vi "Motion_subsystem.vi"(10 "Parameters":dbl[](array[numeric]), 11 "ControlWord":u16 format="%.0b") -> (2 "Results":dbl[](array[numeric]), 3 "StatusWord":u16, 4 "Enum":T1)   [LabVIEW 2017]
uses:
  Utilities/StateMachine.ctl
  SoftmotionAxis/SoftmotionAxis.lvclass
  Utilities/Controlword_Commands.ctl
  Utilities/Mode.ctl
  Utilities/WordManipulationLibrary.lvlib
  Utilities/Bit Manipulation.lvlib
panel:
  out "error out":errorcluster
  in  "error in":errorcluster
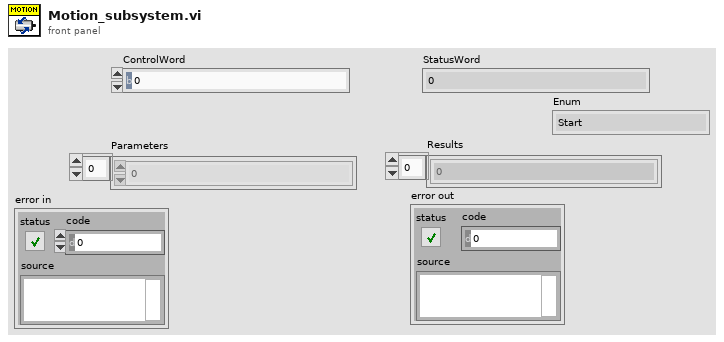
[diagram p1: front panel]
types:
  T1 = typedef "WordManipulationLibrary.lvlib/StateMachine.ctl" = enum16{"Start", "Not Ready to Switch On", "Switch On Disabled", "Ready to Switch On", "Switched On", "Operation enable", "Quick Stop Active", "Fault Reaction Active", "Fault"}
  T2 = typedef "WordManipulationLibrary.lvlib/Controlword_Commands.ctl" = enum16{"Shutdown", "Switch On", "Disable Voltage", "Quick Stop", "Disable Op", "Enable Op", "Fault Reset", "Error"}
  T3 = typedef "WordManipulationLibrary.lvlib/Mode.ctl" = enum16{"Reserved", "Profile Position Mode", "Velocity Mode", "Profile Velocity Mode", "Profile Torque Mode", "Reserved 2", "Reference Mode", "Interpolated Position Mode", "Skip"}
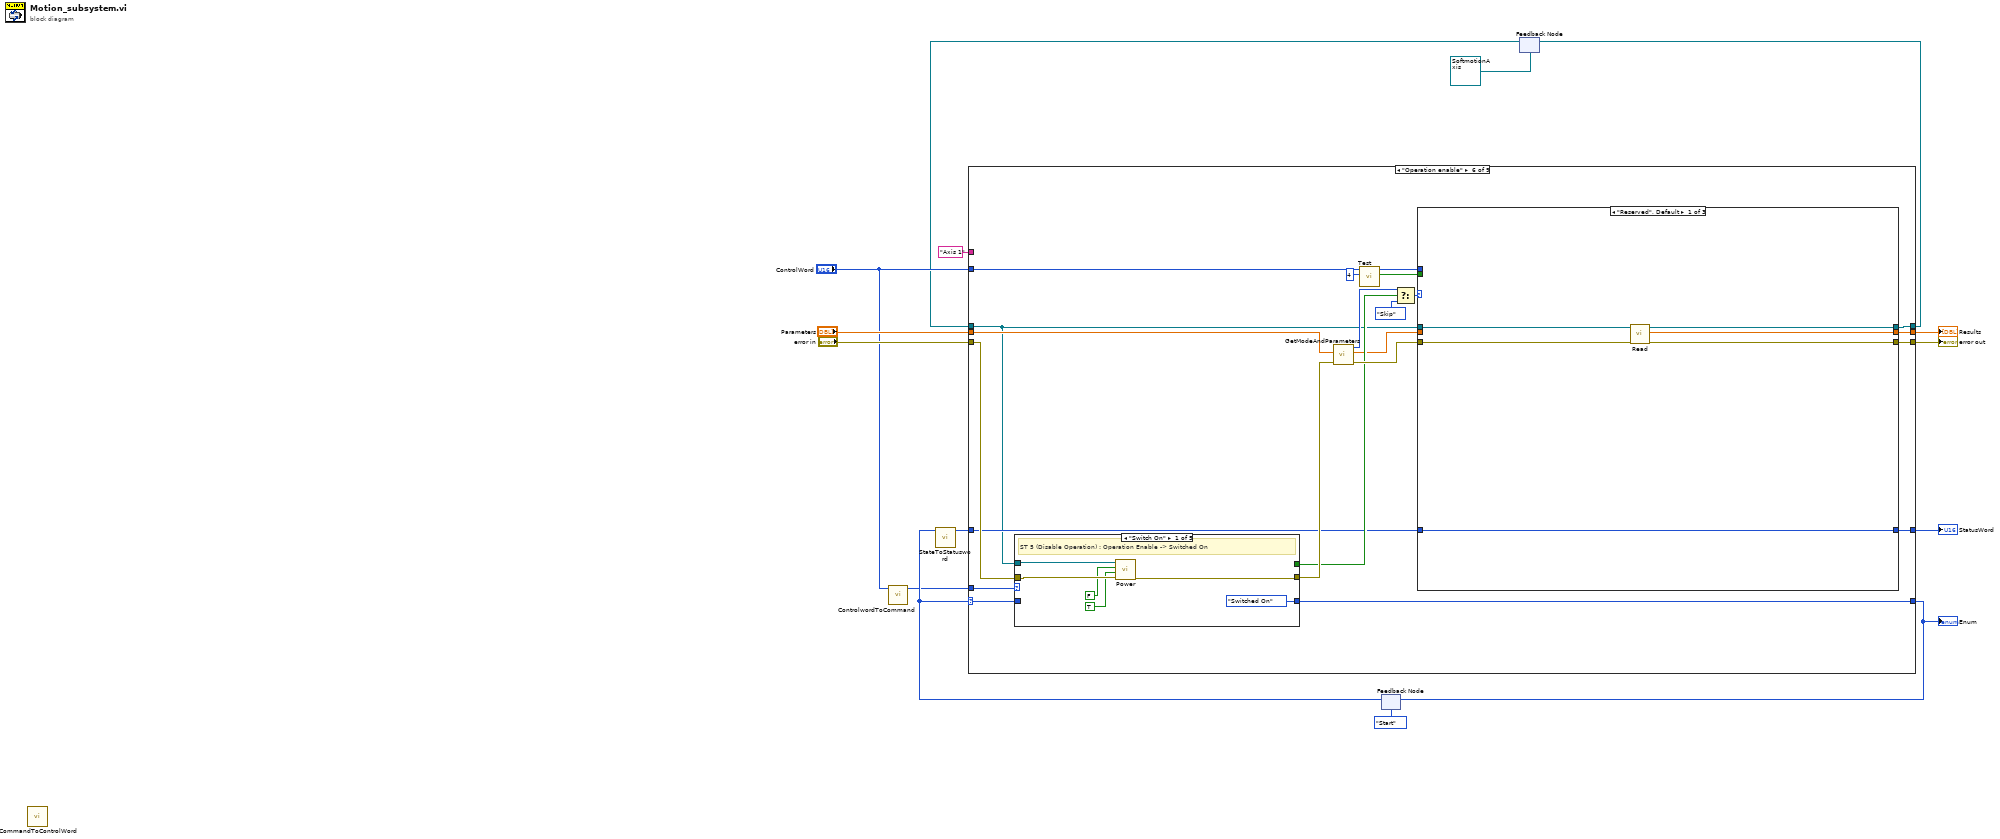
[diagram p0: block diagram]
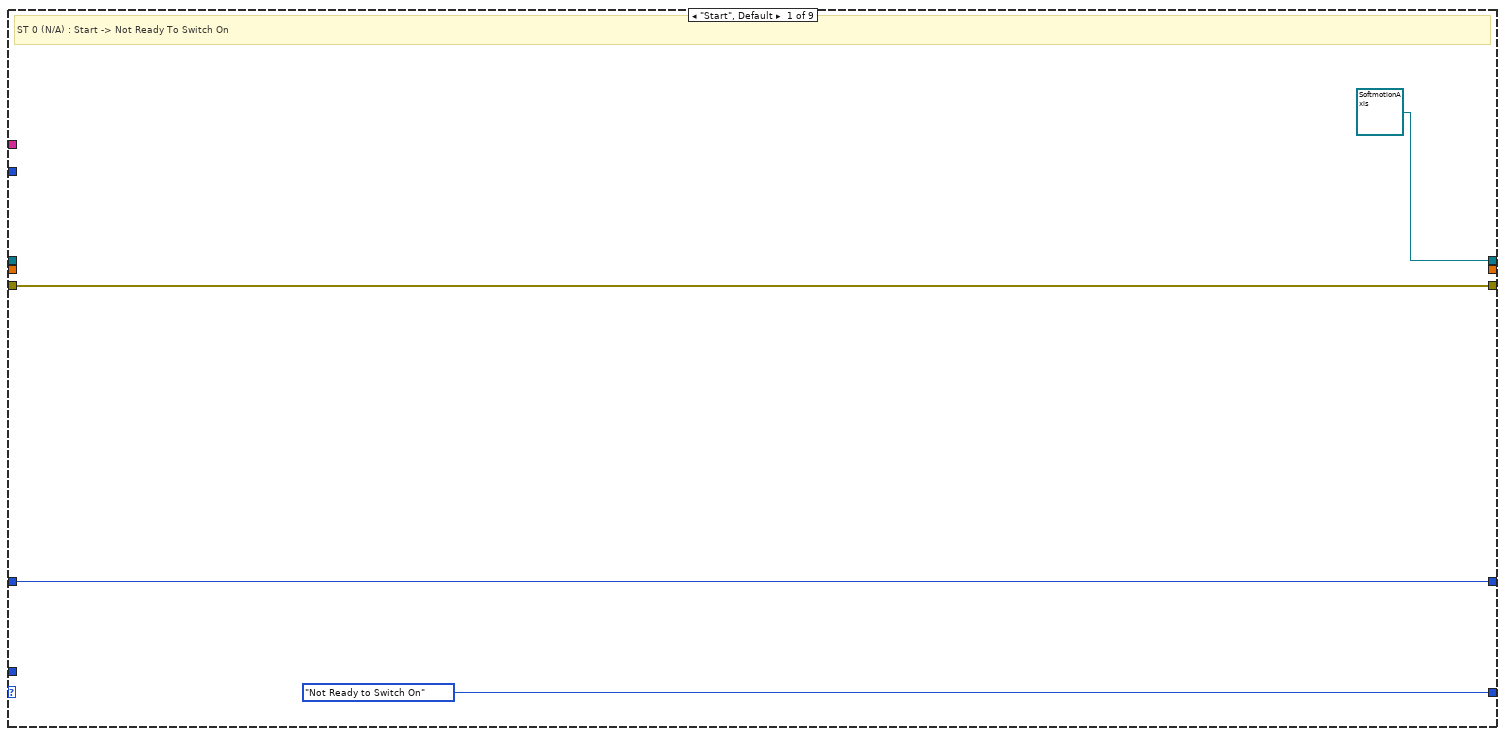
[diagram p2: hidden frame]
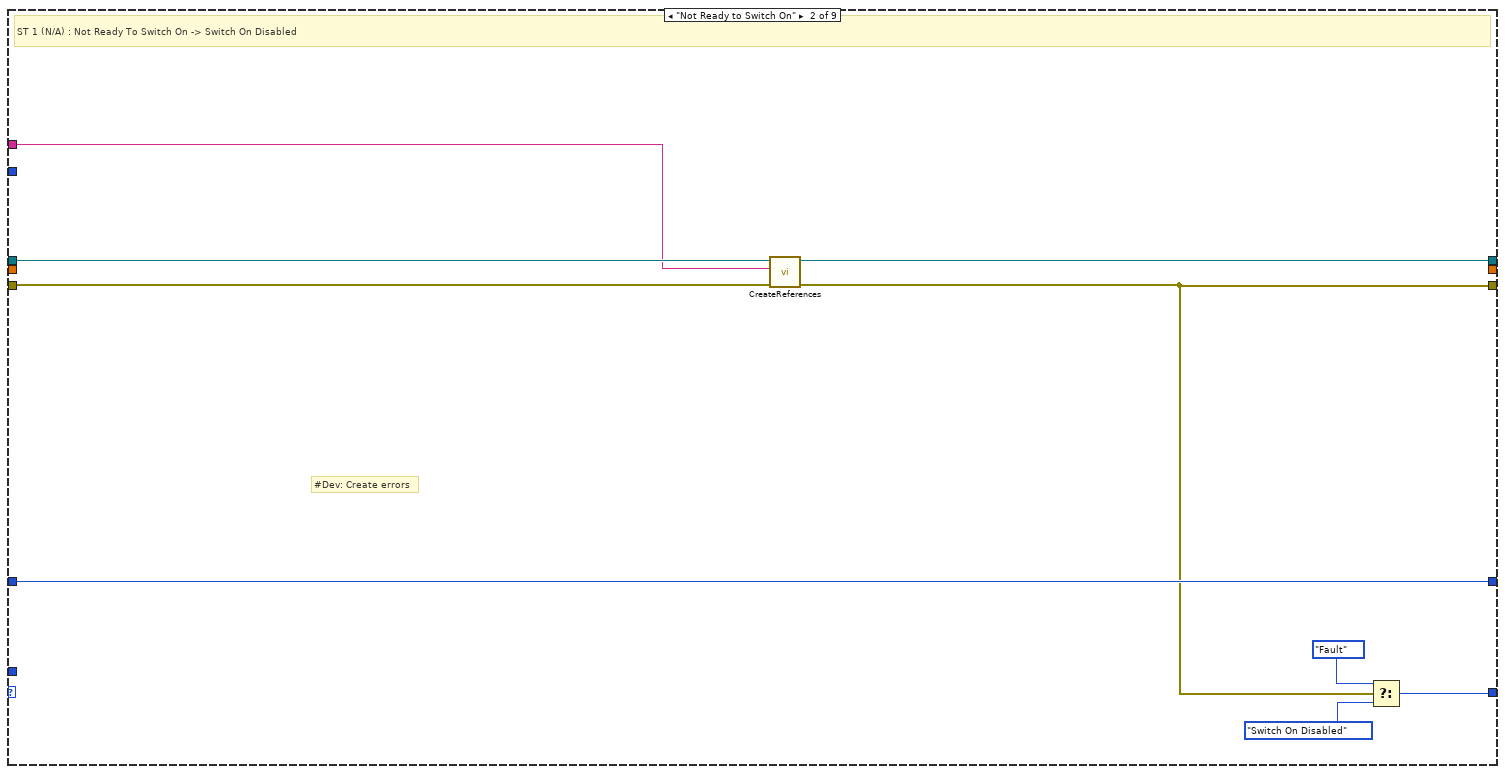
[diagram p3: hidden frame]
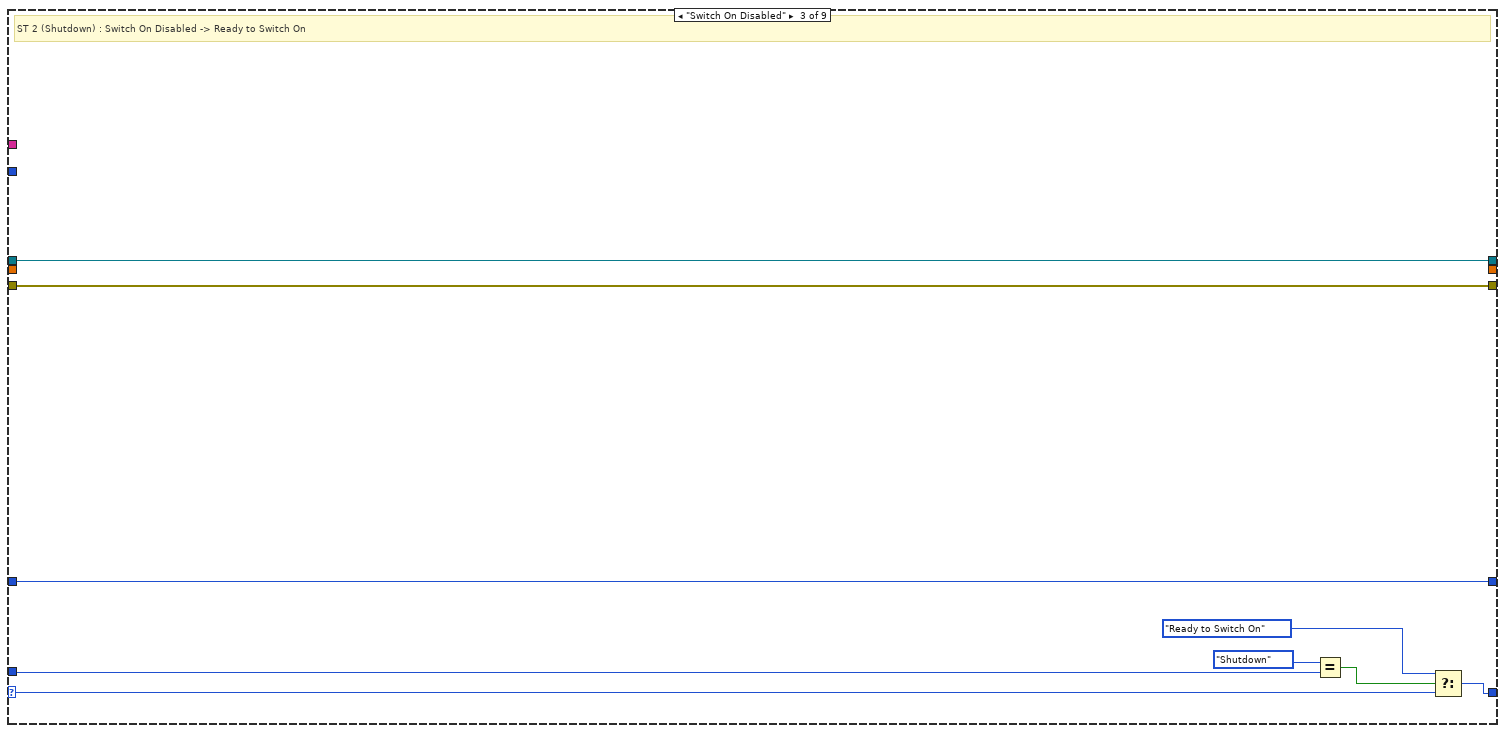
[diagram p4: hidden frame]
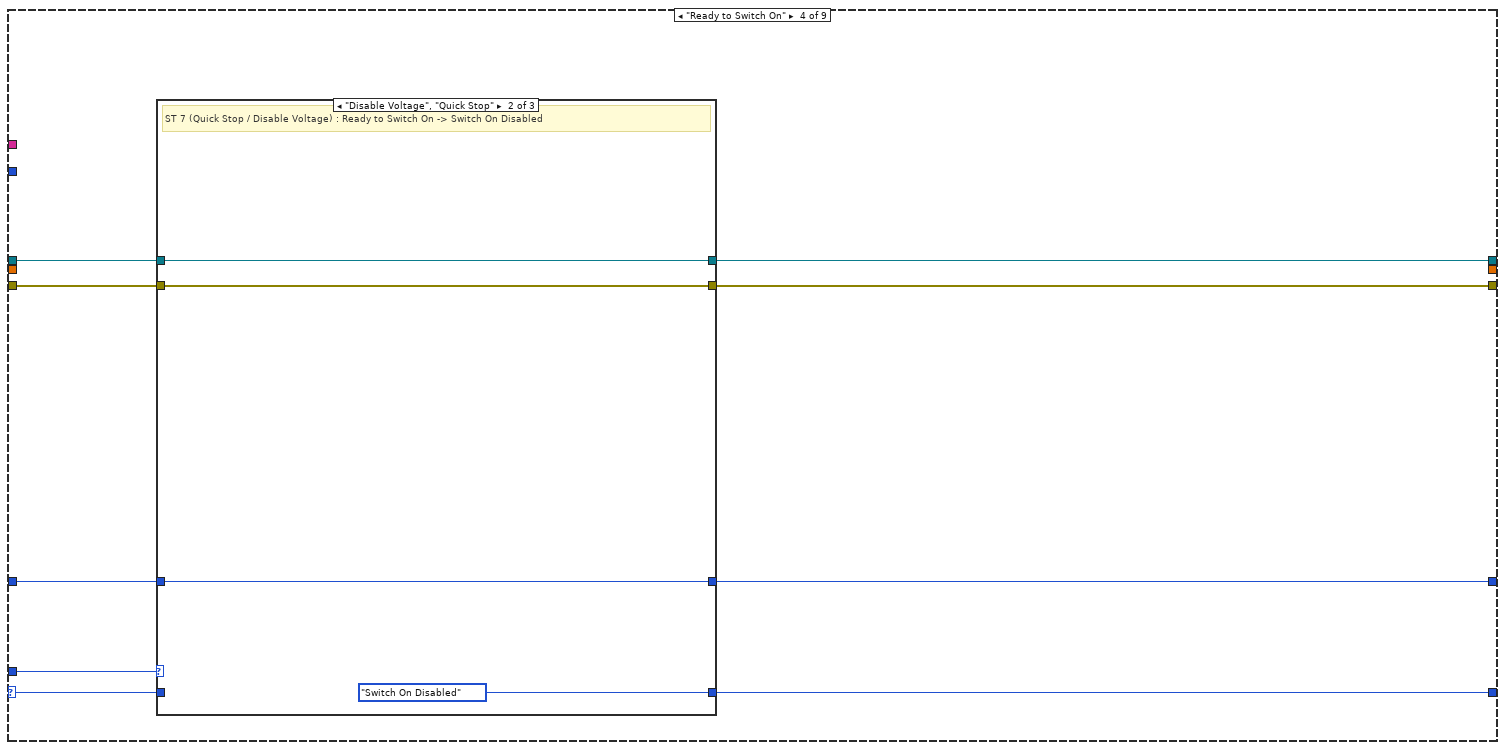
[diagram p5: hidden frame]
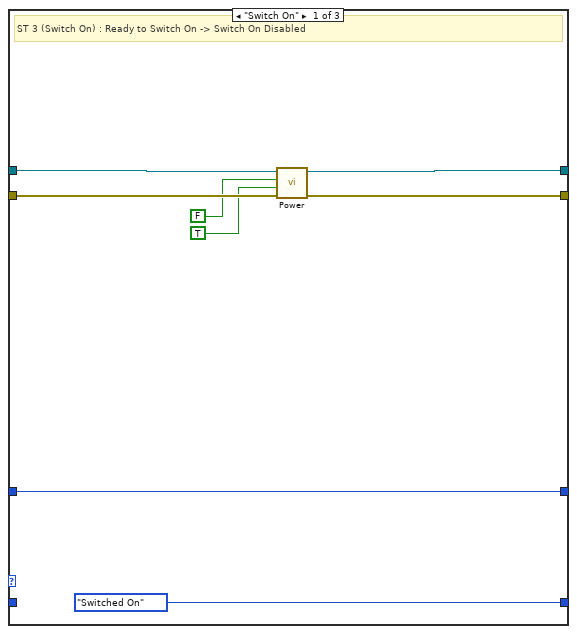
[diagram p6: hidden frame]
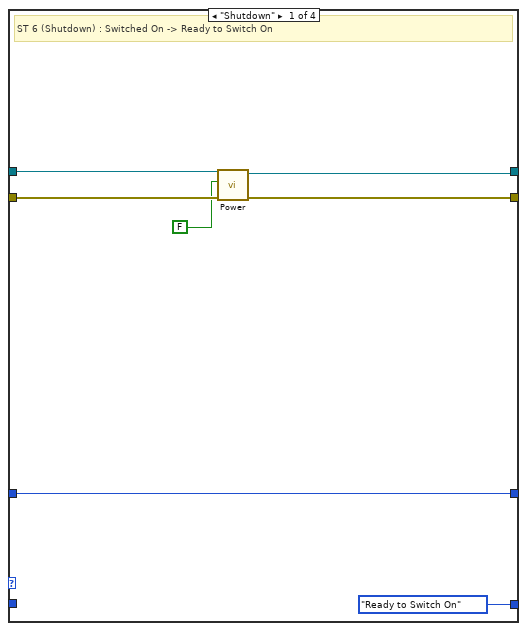
[diagram p9: hidden frame]
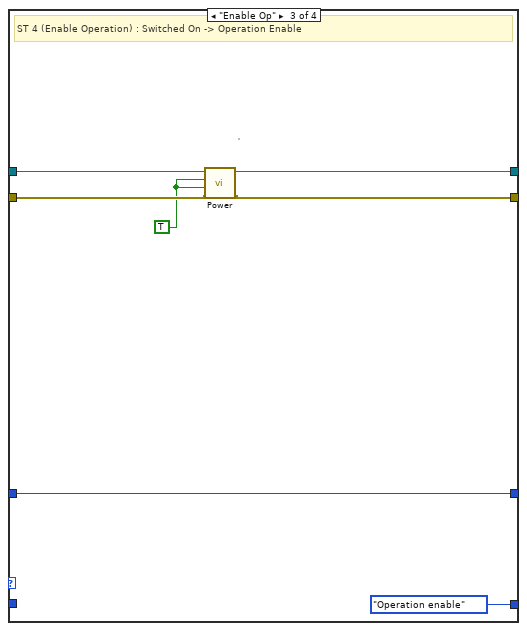
[diagram p10: hidden frame]
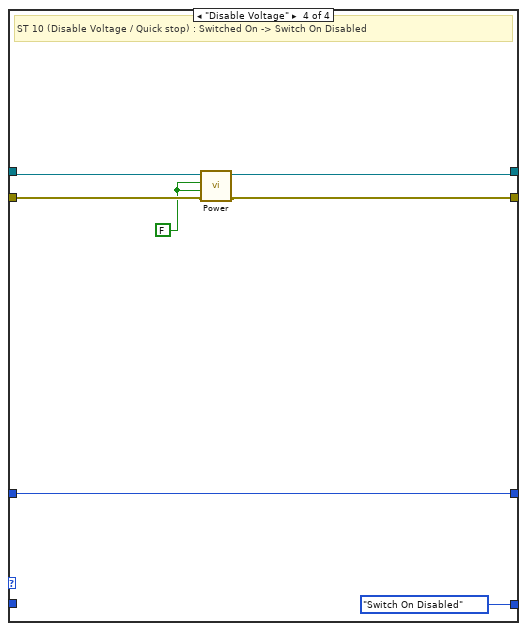
[diagram p11: hidden frame]
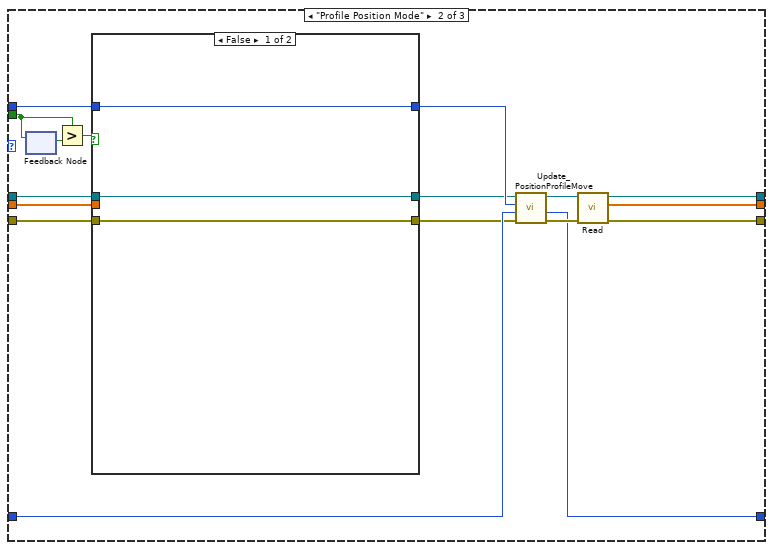
[diagram p12: hidden frame]
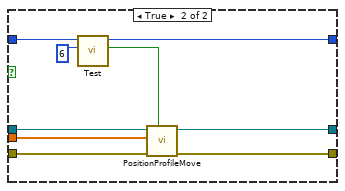
[diagram p13: hidden frame]
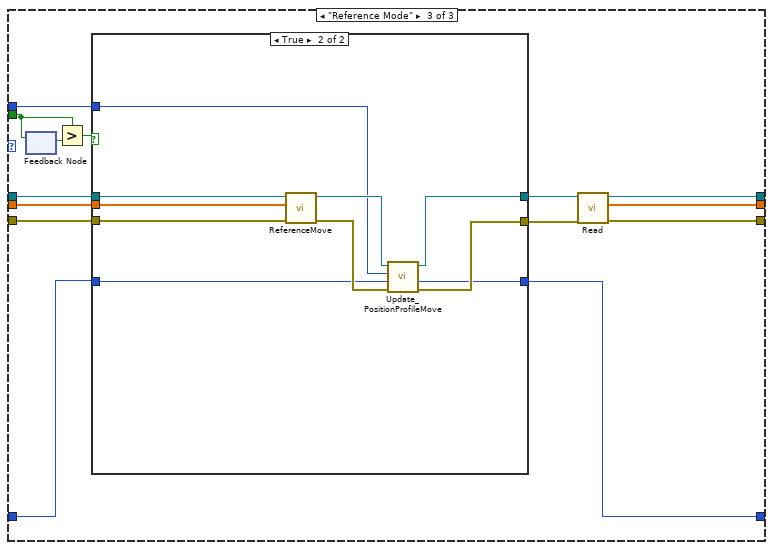
[diagram p14: hidden frame]
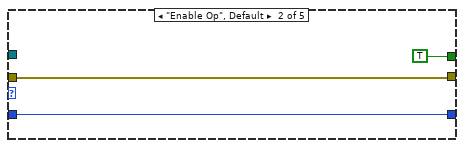
[diagram p16: hidden frame]
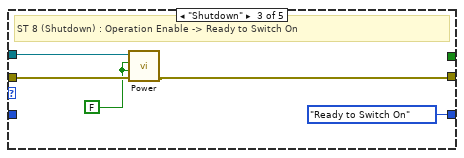
[diagram p17: hidden frame]
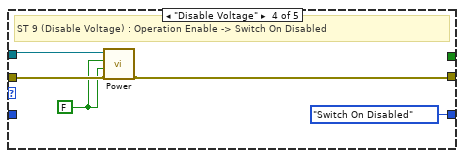
[diagram p18: hidden frame]
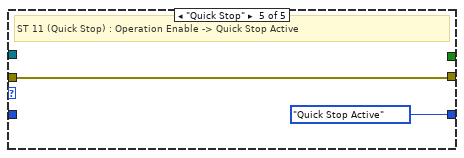
[diagram p19: hidden frame]
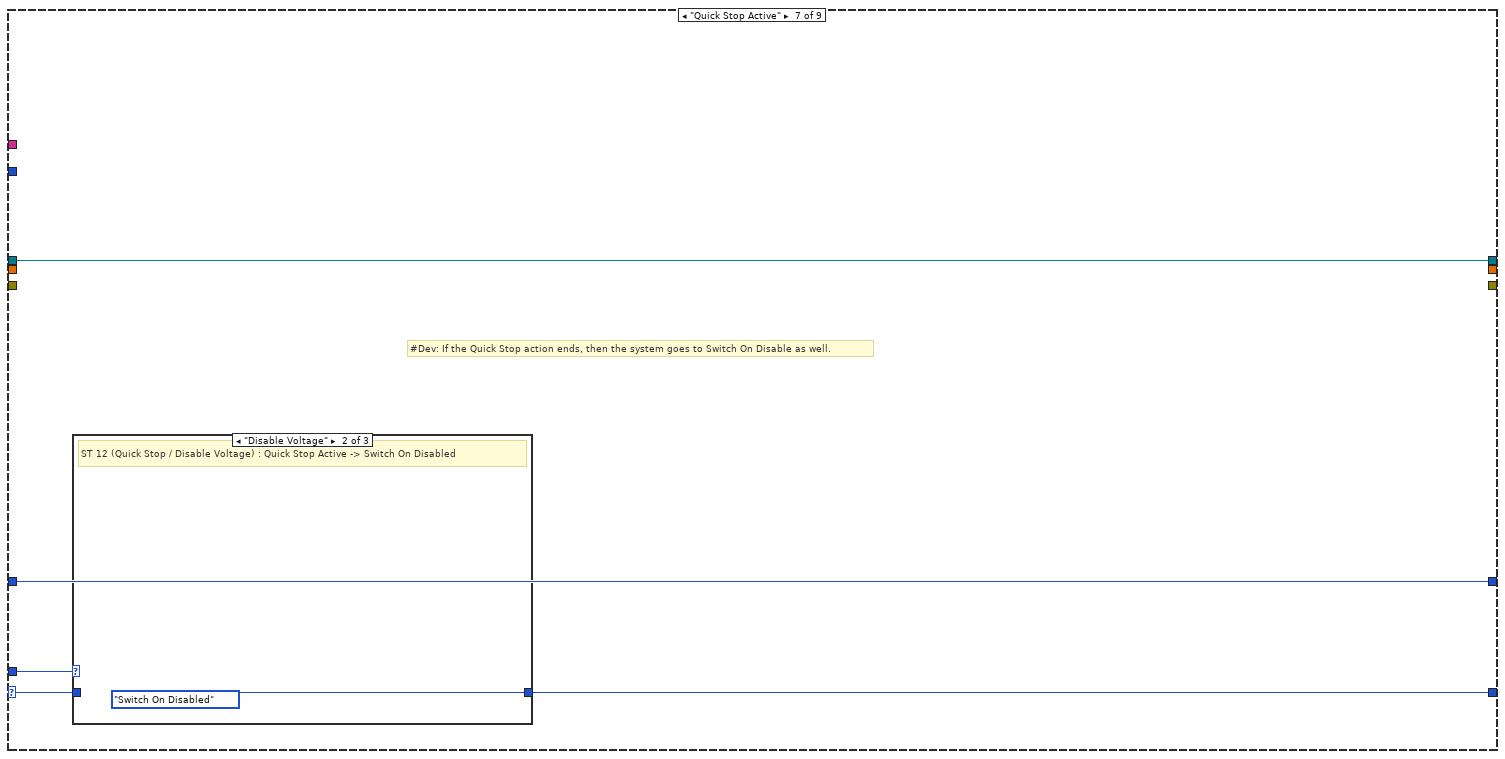
[diagram p20: hidden frame]
diagram:
  n1 = call "CommandToControlWord.vi"() -> ()  [unwired: 11 in, 1 out]
  n2 = call "ControlwordToCommand.vi"("Data_In"="ControlWord") -> ("Device Control Command"=w4:T2)  [unwired: 10 in]
  n3 = feedback #1(StateMachine."Start") -> (w13:T1)
  n4 = call "StateToStatusword.vi"("CurrentStatus"=w13) -> ("StatusWord Out"=w12:u16)  [unwired: 10 in]
  n5 = feedback #2(refnum<class "SoftmotionAxis.lvclass"> refnum ("SoftmotionAxis.lvclass")) -> (w2:refnum<class "SoftmotionAxis.lvclass">)
  n6 = case shown="\"Operation enable\"" w13 {
    selector: w13 -> [_ _ w33 w45 w70 w117 w204 _ w215]
    tunnel: w4 -> [_ _ w37 w46 w71 w118 w206 _ w216]
    tunnel: [StateMachine."Not Ready to Switch On" w25 w32 w44 w69 w116 w205 StateMachine."Fault" w217] -> w14
    tunnel: [w18 w28 w31 w40 w66 w113 w203 w211 w214] -> w11
    tunnel: w12 -> [w18 w28 w31 w41 w67 w102 w203 w211 w214]
    tunnel: "ControlWord" -> [_ _ _ _ _ w115 _ _ _]
    tunnel: "Parameters" -> [_ _ _ _ _ w99 _ _ _]
    tunnel: "Axis 1" -> [_ w20 _ _ _ _ _ _ _]
    tunnel: [_ _ _ _ _ w112 _ _ _] -> w8
    tunnel: "error in" -> [w17 w24 w30 w43 w68 w108 _ _ _]
    tunnel: [w17 w21 w30 w42 w65 w100 _ _ _] -> w6
    tunnel: w2 -> [_ w23 w29 w39 w64 w98 w202 w210 w213]
    tunnel: [refnum<class "SoftmotionAxis.lvclass"> refnum ("SoftmotionAxis.lvclass") w22 w29 w38 w63 w97 w202 w210 w213] -> w1
    frame "Start", Default {
      # "ST 0 (N/A) : Start -> Not Ready To Switch On"
    }
    frame "Not Ready to Switch On" {
      # "#Dev: Create errors"
      # "ST 1 (N/A) : Not Ready To Switch On -> Switch On Disabled"
      n7 = call-dynamic "CreateReferences.vi"("error in (no error)"=w24, "Axis Name"=w20, "SoftmotionAxis in"=w23) -> ("error out"=w21:errorcluster, "SoftmotionAxis out"=w22:refnum<class "SoftmotionAxis.lvclass">)  [unwired: 7 in]
      n8 = Select(t=StateMachine."Fault", s=w21, f=StateMachine."Switch On Disabled") -> (s? t:f=w25:T1)
    }
    frame "Switch On Disabled" {
      # "ST 2 (Shutdown) : Switch On Disabled -> Ready to Switch On"
      n9 = Equal?(x=Controlword_Commands."Shutdown" ("Device Control Command"), y=w37) -> (x = y?=w36:bool)
      n10 = Select(t=StateMachine."Ready to Switch On", s=w36, f=w33) -> (s? t:f=w32:T1)
    }
    frame "Ready to Switch On" {
      n11 = case shown="\"Disable Voltage\", \"Quick Stop\"" w46 {
        tunnel: w45 -> [_ _ w62]
        tunnel: [StateMachine."Switched On" StateMachine."Switch On Disabled" w62] -> w44
        tunnel: w43 -> [w51 w57 w61]
        tunnel: [w52 w57 w61] -> w42
        tunnel: [w53 w56 w60] -> w40
        tunnel: w41 -> [w53 w56 w60]
        tunnel: w39 -> [w50 w55 w59]
        tunnel: [w47 w55 w59] -> w38
        frame "Switch On" {
          # "ST 3 (Switch On) : Ready to Switch On -> Switch On Disabled"
          n12 = call-dynamic "Power.vi"("error in (no error)"=w51, "Enable Drive"=TRUE, "Enable Axis"=FALSE, "SoftmotionAxis in"=w50) -> ("error out"=w52:errorcluster, "SoftmotionAxis out"=w47:refnum<class "SoftmotionAxis.lvclass">)  [unwired: 6 in]
        }
        frame "Disable Voltage", "Quick Stop" {
          # "ST 7 (Quick Stop / Disable Voltage) : Ready to Switch On -> Switch On Disabled"
        }
        frame Default {
          # "No Op."
        }
      }
    }
    frame "Switched On" {
      n13 = case shown="Default" w71 {
        tunnel: w70 -> [_ w82 _ _]
        tunnel: [StateMachine."Ready to Switch On" w82 StateMachine."Operation enable" StateMachine."Switch On Disabled"] -> w69
        tunnel: w68 -> [w76 w81 w87 w94]
        tunnel: [w75 w81 w86 w93] -> w65
        tunnel: [w77 w80 w88 w95] -> w66
        tunnel: w67 -> [w77 w80 w88 w95]
        tunnel: w64 -> [w73 w79 w85 w92]
        tunnel: [w72 w79 w83 w91] -> w63
        frame "Shutdown" {
          # "ST 6 (Shutdown) : Switched On -> Ready to Switch On"
          n14 = call-dynamic "Power.vi"("error in (no error)"=w76, "Enable Axis"=FALSE, "SoftmotionAxis in"=w73) -> ("error out"=w75:errorcluster, "SoftmotionAxis out"=w72:refnum<class "SoftmotionAxis.lvclass">)  [unwired: 7 in]
        }
        frame Default {
          # "No op"
        }
        frame "Enable Op" {
          w84 = TRUE ("Enable Axis")
          # "ST 4 (Enable Operation) : Switched On -> Operation Enable"
          n15 = call-dynamic "Power.vi"("error in (no error)"=w87, "Enable Drive"=w84, "Enable Axis"=w84, "SoftmotionAxis in"=w85) -> ("error out"=w86:errorcluster, "SoftmotionAxis out"=w83:refnum<class "SoftmotionAxis.lvclass">)  [unwired: 6 in]
        }
        frame "Disable Voltage" {
          w90 = FALSE ("Enable Axis")
          # "ST 10 (Disable Voltage / Quick stop) : Switched On -> Switch On Disabled"
          n16 = call-dynamic "Power.vi"("error in (no error)"=w94, "Enable Drive"=w90, "Enable Axis"=w90, "SoftmotionAxis in"=w92) -> ("error out"=w93:errorcluster, "SoftmotionAxis out"=w91:refnum<class "SoftmotionAxis.lvclass">)  [unwired: 6 in]
        }
      }
    }
    frame "Operation enable" {
      n17 = case shown="\"Switch On\"" w118 {
        tunnel: w117 -> [_ w189 _ _ _]
        tunnel: [StateMachine."Switched On" w189 StateMachine."Ready to Switch On" StateMachine."Switch On Disabled" StateMachine."Quick Stop Active"] -> w116
        tunnel: w108 -> [w185 w188 w193 w198 w200]
        tunnel: [w184 w188 w192 w197 w200] -> w107
        tunnel: [_ TRUE _ _ _] -> w104
        tunnel: w98 -> [w183 _ w190 w195 _]
        frame "Switch On" {
          # "ST 5 (Disable Operation) : Operation Enable -> Switched On"
          n18 = call-dynamic "Power.vi"("error in (no error)"=w185, "Enable Drive"=TRUE, "Enable Axis"=FALSE, "SoftmotionAxis in"=w183) -> ("error out"=w184:errorcluster)  [unwired: 6 in, 1 out]
        }
        frame "Enable Op", Default {
        }
        frame "Shutdown" {
          w191 = FALSE ("Enable Axis")
          # "ST 8 (Shutdown) : Operation Enable -> Ready to Switch On"
          n19 = call-dynamic "Power.vi"("error in (no error)"=w193, "Enable Drive"=w191, "Enable Axis"=w191, "SoftmotionAxis in"=w190) -> ("error out"=w192:errorcluster)  [unwired: 6 in, 1 out]
        }
        frame "Disable Voltage" {
          w196 = FALSE ("Enable Axis")
          # "ST 9 (Disable Voltage) : Operation Enable -> Switch On Disabled"
          n20 = call-dynamic "Power.vi"("error in (no error)"=w198, "Enable Drive"=w196, "Enable Axis"=w196, "SoftmotionAxis in"=w195) -> ("error out"=w197:errorcluster)  [unwired: 6 in, 1 out]
        }
        frame "Quick Stop" {
          # "ST 11 (Quick Stop) : Operation Enable -> Quick Stop Active"
        }
      }
      n21 = call "GetModeAndParameters.vi"("error in (no error)"=w107, "Parameters"=w99) -> ("error out"=w109:errorcluster, "Parameters Out"=w101:dbl[], "f"=w106:T3)  [unwired: 7 in]
      n22 = call "Test.vi"("Bit to test"=u8 4, "Data_In"=w115) -> ("bit value"=w110:bool, "Data_Out"=w111:u16)  [unwired: 8 in]
      n23 = Select(t=w106, s=w104, f=Mode."Skip") -> (s? t:f=w105:T3)
      n24 = case shown="\"Reserved\", Default" w105 {
        tunnel: w110 -> [_ w138 w164]
        tunnel: [w124 w128 w160] -> w113
        tunnel: w102 -> [w124 w135 w161]
        tunnel: [w123 w133 w158] -> w112
        tunnel: w111 -> [_ w141 w167]
        tunnel: w101 -> [_ w139 w165]
        tunnel: w109 -> [w121 w140 w166]
        tunnel: [w122 w132 w156] -> w100
        tunnel: w98 -> [w120 w134 w159]
        tunnel: [w119 w131 w154] -> w97
        frame "Reserved", Default {
          n25 = call-dynamic "Read.vi"("error in (no error)"=w121, "SoftmotionAxis in"=w120) -> ("error out"=w122:errorcluster, "appended array"=w123:dbl[], "SoftmotionAxis out"=w119:refnum<class "SoftmotionAxis.lvclass">)  [unwired: 7 in]
        }
        frame "Profile Position Mode" {
          n26 = feedback-in #3(w138) -> ()
          n27 = feedback #3() -> (w137:bool)  [unwired: 1 in]
          n28 = Greater?(x=w138, y=w137) -> (0:w136:bool)
          n29 = case shown="False" w136 {
            tunnel: w141 -> [w142 w153]
            tunnel: w140 -> [w143 w151]
            tunnel: w139 -> [_ w150]
            tunnel: w134 -> [w144 w148]
            tunnel: [w144 w145] -> w125
            tunnel: [w142 w147] -> w130
            tunnel: [w143 w146] -> w126
            frame False {
            }
            frame True {
              n30 = call "Test.vi"("Bit to test"=u8 6, "Data_In"=w153) -> ("bit value"=w149:bool, "Data_Out"=w147:u16)  [unwired: 8 in]
              n31 = call-dynamic "PositionProfileMove.vi"("Relative?"=w149, "error in (no error)"=w151, "Array"=w150, "SoftmotionAxis in"=w148) -> ("error out"=w146:errorcluster, "SoftmotionAxis out"=w145:refnum<class "SoftmotionAxis.lvclass">)  [unwired: 6 in]
            }
          }
          n32 = call-dynamic "Update_PositionProfileMove.vi"("error in (no error)"=w126, "StatusWord"=w135, "ControlWord"=w130, "SoftmotionAxis in"=w125) -> ("error out"=w129:errorcluster, "StatusWord Out"=w128:u16, "SoftmotionAxis out"=w127:refnum<class "SoftmotionAxis.lvclass">)  [unwired: 5 in]
          n33 = call-dynamic "Read.vi"("error in (no error)"=w129, "SoftmotionAxis in"=w127) -> ("error out"=w132:errorcluster, "appended array"=w133:dbl[], "SoftmotionAxis out"=w131:refnum<class "SoftmotionAxis.lvclass">)  [unwired: 7 in]
        }
        frame "Reference Mode" {
          n34 = feedback-in #4(w164) -> ()
          n35 = feedback #4() -> (w163:bool)  [unwired: 1 in]
          n36 = Greater?(x=w164, y=w163) -> (0:w162:bool)
          n37 = case shown="True" w162 {
            tunnel: w167 -> [_ w171]
            tunnel: w166 -> [w170 w180]
            tunnel: w165 -> [_ w179]
            tunnel: [w170 w177] -> w157
            tunnel: w161 -> [w169 w173]
            tunnel: [w169 w176] -> w160
            tunnel: w159 -> [w168 w178]
            tunnel: [w168 w172] -> w155
            frame False {
            }
            frame True {
              n38 = call-dynamic "ReferenceMove.vi"("error in (no error)"=w180, "Array"=w179, "SoftmotionAxis in"=w178) -> ("error out"=w174:errorcluster, "SoftmotionAxis out"=w175:refnum<class "SoftmotionAxis.lvclass">)  [unwired: 7 in]
              n39 = call-dynamic "Update_PositionProfileMove.vi"("error in (no error)"=w174, "StatusWord"=w173, "ControlWord"=w171, "SoftmotionAxis in"=w175) -> ("error out"=w177:errorcluster, "StatusWord Out"=w176:u16, "SoftmotionAxis out"=w172:refnum<class "SoftmotionAxis.lvclass">)  [unwired: 5 in]
            }
          }
          n40 = call-dynamic "Read.vi"("error in (no error)"=w157, "SoftmotionAxis in"=w155) -> ("error out"=w156:errorcluster, "appended array"=w158:dbl[], "SoftmotionAxis out"=w154:refnum<class "SoftmotionAxis.lvclass">)  [unwired: 7 in]
        }
      }
    }
    frame "Quick Stop Active" {
      # "#Dev: If the Quick Stop action ends, then the system goes to Switch On Disable as well."
      n41 = case shown="\"Disable Voltage\"" w206 {
        tunnel: w204 -> [_ _ w209]
        tunnel: [StateMachine."Operation enable" StateMachine."Switch On Disabled" w209] -> w205
        frame "Enable Op" {
          # "ST 16 (Enable Operation) : Quick Stop Active -> Operation Enable"
        }
        frame "Disable Voltage" {
          # "ST 12 (Quick Stop / Disable Voltage) : Quick Stop Active -> Switch On Disabled"
        }
        frame "Shutdown", Default {
          # "No Transition"
        }
      }
    }
    frame "Fault Reaction Active" {
      # "#Dev: Add transition ST 15 (Fault Reset) : Fault Reaction Active -> Switch On Disabled"
      # "#Dev: Deal with Fault here (Log, communicate, etc)"
      # "ST 14 (N/A) : Fault Reaction Active -> Fault"
    }
    frame "Fault" {
      n42 = case shown="\"Shutdown\", Default" w216 {
        tunnel: [w218 StateMachine."Switch On Disabled"] -> w217
        tunnel: w215 -> [w218 _]
        frame "Shutdown", Default {
        }
        frame "Fault Reset" {
        }
      }
    }
  }
  "StatusWord" <- w11
  "Results" <- w8
  "Enum" <- w14
  "error out" <- w6
  n43 = feedback-in #1(w14) -> ()
  n44 = feedback-in #2(w1) -> ()
